vi "ABB measure Temperature.vi"(10 "Simulate":bool, 11 "Mode":enum16{"Initialise", "Read", "Close"}(ring)) -> (0 "error out":errorcluster, 2 "Reading strings":string[](array[string]), 3 "Readings":dbl[](array[numeric]))   [LabVIEW 2017]
uses:
  RTD Type.ctl
  TC Type.ctl
  <vilib>/DAQmx/read.llb/DAQmx Read (Analog 2D DBL NChan NSamp).vi
  <vilib>/Analysis/baseanly.llb/Mean (DBL).vi
  ABB global.vi
  <vilib>/DAQmx/create/channels.llb/DAQmx Create Channel (AI-Temperature-RTD).vi
  <vilib>/DAQmx/configure/timing.llb/DAQmx Timing (Sample Clock).vi
  <vilib>/DAQmx/create/channels.llb/DAQmx Create Channel (AI-Temperature-Thermocouple).vi
  <vilib>/DAQmx/miscellaneous.llb/DAQmx Fill In Error Info.vi
  <resource>/objmgr/daqmx.rc
  <vilib>/Analysis/NI_AALBase.lvlib
panel:
  out "error out 2":errorcluster
  out "AvailSampPerChan":u32
  out "RT resistance":dbl[](array[numeric])
  out "RT types":i32[](array[numeric])
  out "TC Types":i32[](array[numeric])
  in  "Thermocouple Type":T1 items=["J", "K", "N", "R", "S", "T", "B", "E"]
  in  "RTD Type":T2 items=["PT100 3W", "PT100 4W", "PT1000 3W", "PT1000 4W"]
  out "Array":string[](array[string])
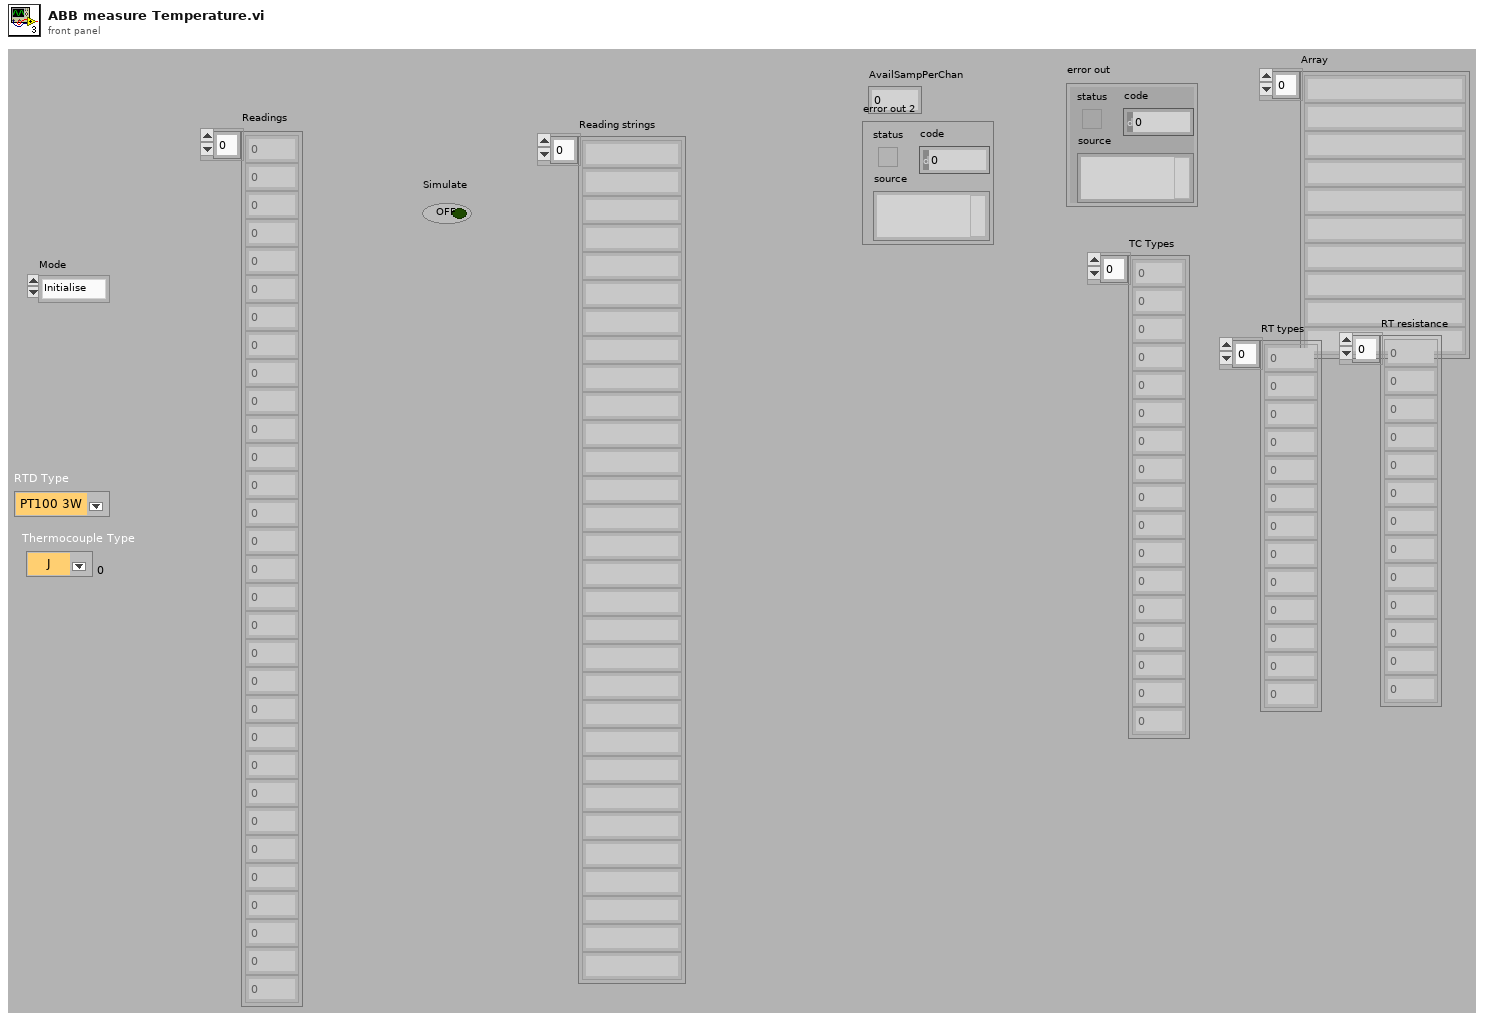
[diagram p1: front panel]
types:
  T1 = typedef "TC Type.ctl" = u16
  T2 = typedef "RTD Type.ctl" = u16
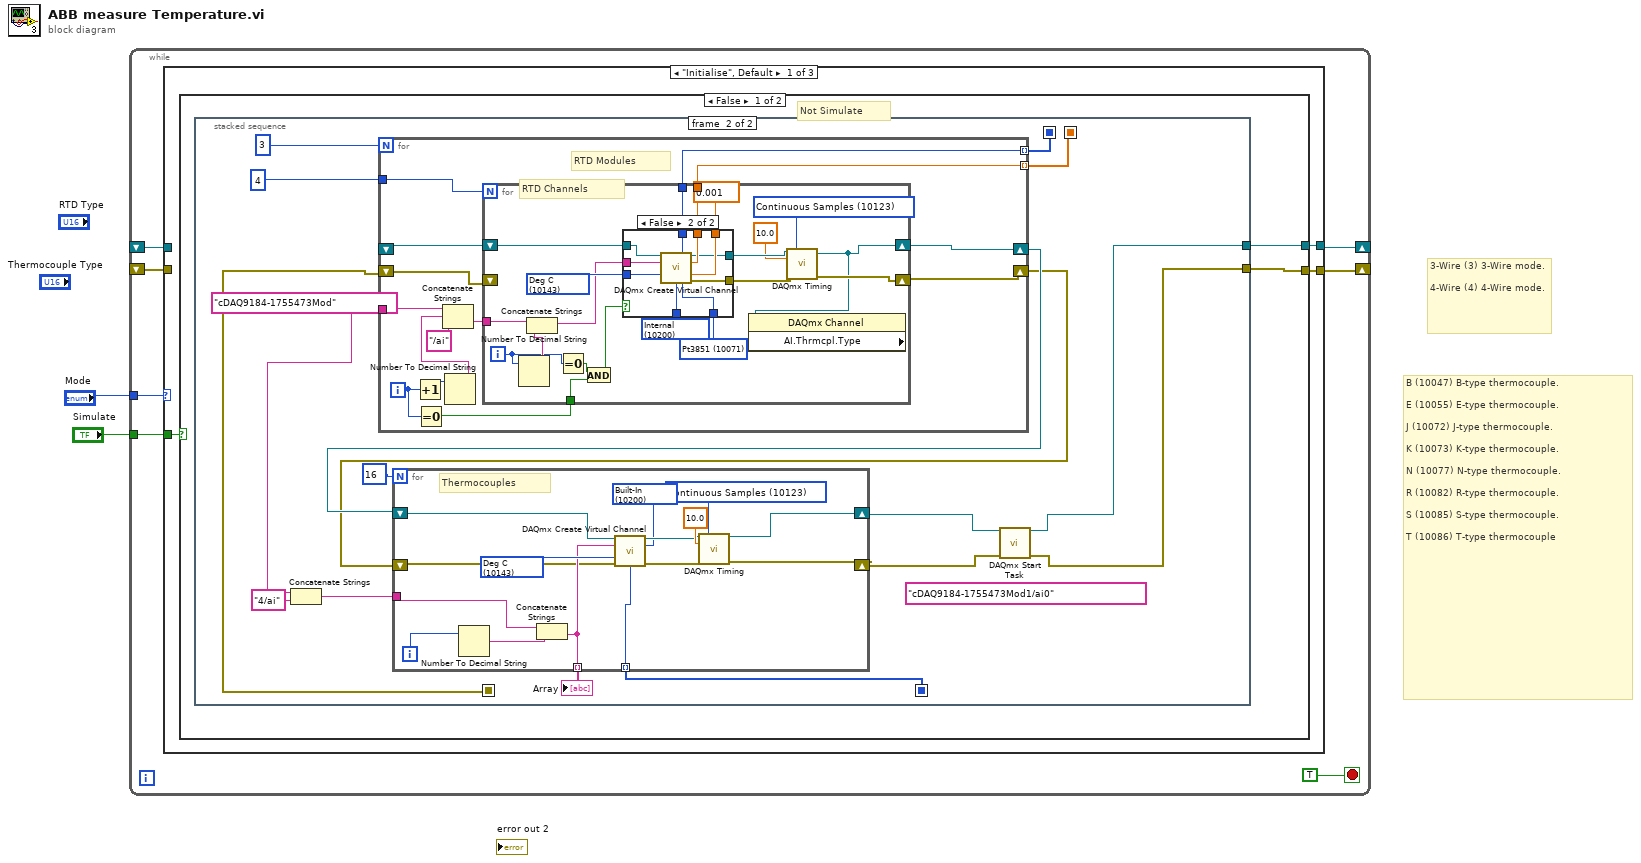
[diagram p0: block diagram]
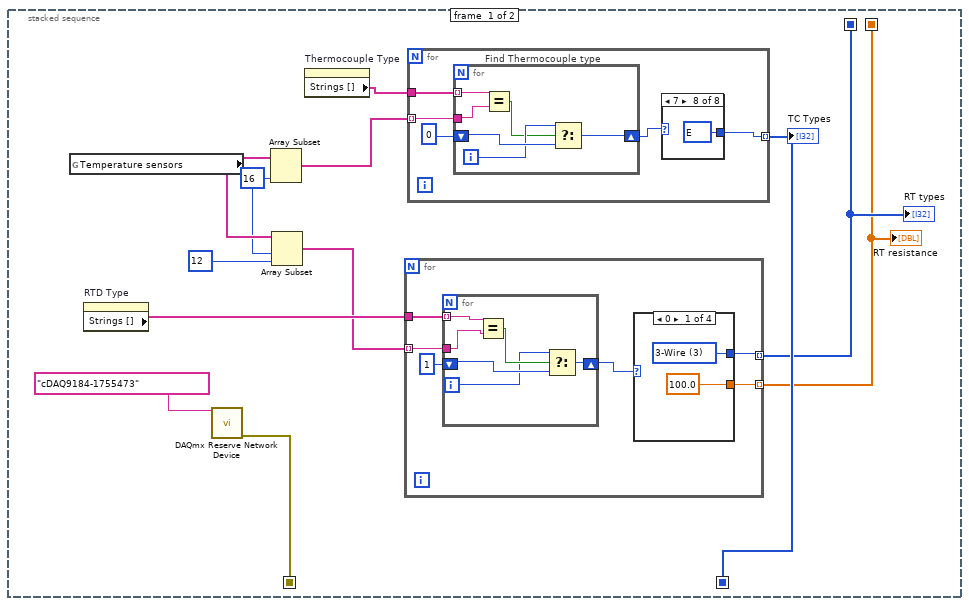
[diagram p2: hidden frame]
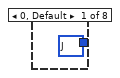
[diagram p3: hidden frame]
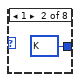
[diagram p4: hidden frame]
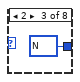
[diagram p5: hidden frame]
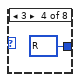
[diagram p6: hidden frame]
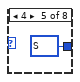
[diagram p7: hidden frame]
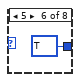
[diagram p8: hidden frame]
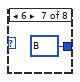
[diagram p9: hidden frame]
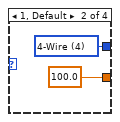
[diagram p10: hidden frame]
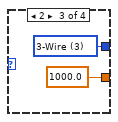
[diagram p11: hidden frame]
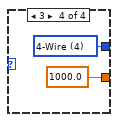
[diagram p12: hidden frame]
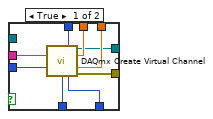
[diagram p13: hidden frame]
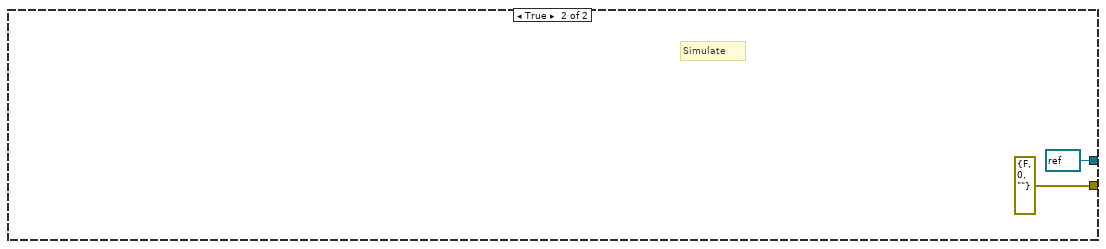
[diagram p14: hidden frame]
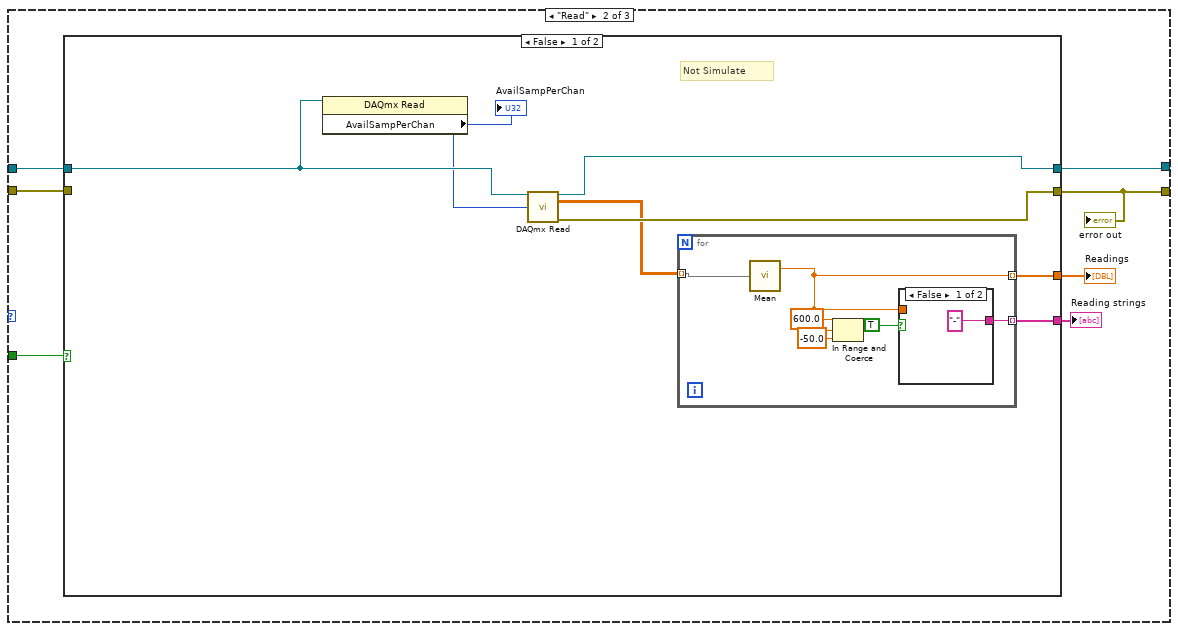
[diagram p15: hidden frame]
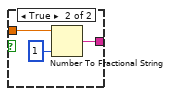
[diagram p16: hidden frame]
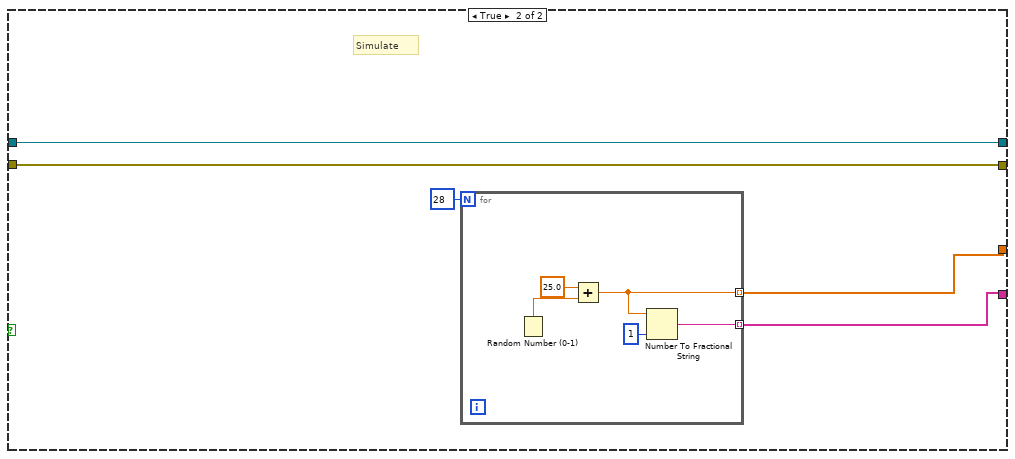
[diagram p17: hidden frame]
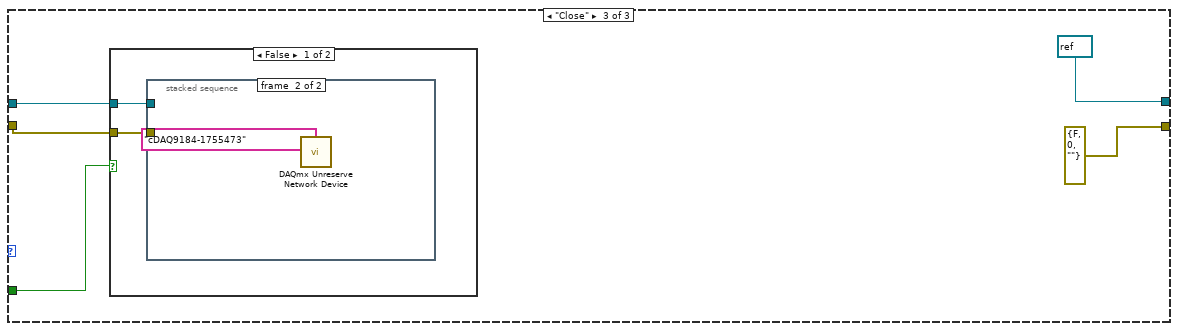
[diagram p18: hidden frame]
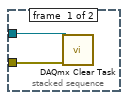
[diagram p19: hidden frame]
diagram:
  # "3-Wire (3) 3-Wire mode. \n \n4-Wire (4) 4-Wire mode."
  # "B (10047) B-type thermocouple. \n \nE (10055) E-type thermocouple. \n \nJ (10072) J-type thermocouple. \n \nK (10073) K-type thermocouple. \n \nN (10077) N-type thermocouple. \n \nR (10082) R-type thermocouple. \n \nS (10085) S-type thermocouple. \n \nT (10086) T-type thermocouple"
  n1 = while {
    tunnel: "Mode" -> [w9]
    shift-right: [w4] -> _
    shift-left: _ -> [w7]
    shift-right: [w5] -> _
    shift-left: _ -> [w6]
    tunnel: "Simulate" -> [w3]
    stop <- TRUE stop-if-true
    n2 = case shown="\"Initialise\", Default" w9 {
      tunnel: [w12 w159 refnum<k21> refnum ("task out")] -> w4
      tunnel: [w11 w154 errorcluster {"status"=FALSE, "code"=0, "source"=""} ("error out")] -> w5
      tunnel: w7 -> [_ w158 w191]
      tunnel: w6 -> [_ w157 w188]
      tunnel: w3 -> [w10 w156 w187]
      frame "Initialise", Default {
        n3 = case shown="False" w10 {
          tunnel: [w14 refnum<k21> refnum ("task out")] -> w12
          tunnel: [w13 errorcluster {"status"=FALSE, "code"=0, "source"=""} ("error out")] -> w11
          frame False {
            # "Not Simulate"
            n4 = stacked-sequence {
              seq-local: [w21 _] -> [_ w66]
              seq-local: [w18 _] -> [_ w72]
              seq-local: [w17 _] -> [_ w73]
              seq-local: [w15 _] -> [_ w67]
              tunnel: [_ w68] -> w14
              tunnel: [_ w69] -> w13
              frame #0 {
                w25 = 16 ("length")
                n5 = global read "ABB global.vi" "Temperature sensors"() -> (w26:string[])
                n6 = property on="RTD Type" class="Ring (strict)"() -> ("Strings []"=w20:string[])  [unwired: 2 in, 2 out]
                n7 = call <vilib>:"DAQmx Reserve Network Device.vi"("device in"=tag "cDAQ9184-1755473") -> ("error out"=w15:errorcluster)  [unwired: 13 in, 1 out]
                n8 = Array Subset(array=w26, length=w25) -> (w23:string[])  [unwired: 1 in]
                n9 = Array Subset(array=w26, index=w25, length=12) -> (w19:string[])
                n10 = property on="Thermocouple Type" class="Ring (strict)"() -> ("Strings []"=w22:string[])  [unwired: 2 in, 2 out]
                n11 = for {
                  tunnel: w20 -> [w51]
                  tunnel: w19 -> [w50] mode=indexing
                  tunnel: [w48] -> w18 mode=indexing
                  tunnel: [w47] -> w17 mode=indexing
                  n12 = for {
                    tunnel: w51 -> [w64] mode=indexing
                    tunnel: w50 -> [w63]
                    shift-right: [w61] -> w49
                    shift-left: 1 -> [w62]
                    i -> [w60]
                    n13 = Equal?(x=w64, y=w63) -> (x = y?=w65:bool)
                    n14 = Select(t=w60, s=w65, f=w62) -> (s? t:f=w61:i32)
                  }
                  n15 = case shown="0" w49 {
                    tunnel: [w53 w55 w57 w59] -> w48
                    tunnel: [100.0 100.0 1000.0 1000.0] -> w47
                    frame 0 {
                      w53 = 3 items=["2-Wire"=2, "3-Wire"=3, "4-Wire"=4] ("resistance configuration")
                    }
                    frame 1, Default {
                      w55 = 4 items=["2-Wire"=2, "3-Wire"=3, "4-Wire"=4] ("resistance configuration")
                    }
                    frame 2 {
                      w57 = 3 items=["2-Wire"=2, "3-Wire"=3, "4-Wire"=4] ("resistance configuration")
                    }
                    frame 3 {
                      w59 = 4 items=["2-Wire"=2, "3-Wire"=3, "4-Wire"=4] ("resistance configuration")
                    }
                  }
                }
                "RT types" <- w18
                "RT resistance" <- w17
                n16 = for {
                  tunnel: w23 -> [w30] mode=indexing
                  tunnel: w22 -> [w31]
                  tunnel: [w27] -> w21 mode=indexing
                  # "Find Thermocouple type"
                  n17 = for {
                    tunnel: w31 -> [w45] mode=indexing
                    tunnel: w30 -> [w44]
                    shift-right: [w40] -> w28
                    shift-left: 0 -> [w43]
                    i -> [w42]
                    n18 = Equal?(x=w45, y=w44) -> (x = y?=w41:bool)
                    n19 = Select(t=w42, s=w41, f=w43) -> (s? t:f=w40:i32)
                  }
                  n20 = case shown="7" w28 {
                    tunnel: [w32 w33 w34 w35 w36 w37 w38 w39] -> w27
                    frame 0, Default {
                      w32 = 10072 items=["J"=10072, "K"=10073, "N"=10077, "R"=10082, "S"=10085, "T"=10086, "B"=10047, "E"=10055] ("thermocouple type")
                    }
                    frame 1 {
                      w33 = 10073 items=["J"=10072, "K"=10073, "N"=10077, "R"=10082, "S"=10085, "T"=10086, "B"=10047, "E"=10055] ("thermocouple type")
                    }
                    frame 2 {
                      w34 = 10077 items=["J"=10072, "K"=10073, "N"=10077, "R"=10082, "S"=10085, "T"=10086, "B"=10047, "E"=10055] ("thermocouple type")
                    }
                    frame 3 {
                      w35 = 10082 items=["J"=10072, "K"=10073, "N"=10077, "R"=10082, "S"=10085, "T"=10086, "B"=10047, "E"=10055] ("thermocouple type")
                    }
                    frame 4 {
                      w36 = 10085 items=["J"=10072, "K"=10073, "N"=10077, "R"=10082, "S"=10085, "T"=10086, "B"=10047, "E"=10055] ("thermocouple type")
                    }
                    frame 5 {
                      w37 = 10086 items=["J"=10072, "K"=10073, "N"=10077, "R"=10082, "S"=10085, "T"=10086, "B"=10047, "E"=10055] ("thermocouple type")
                    }
                    frame 6 {
                      w38 = 10047 items=["J"=10072, "K"=10073, "N"=10077, "R"=10082, "S"=10085, "T"=10086, "B"=10047, "E"=10055] ("thermocouple type")
                    }
                    frame 7 {
                      w39 = 10055 items=["J"=10072, "K"=10073, "N"=10077, "R"=10082, "S"=10085, "T"=10086, "B"=10047, "E"=10055] ("thermocouple type")
                    }
                  }
                }
                "TC Types" <- w21
              }
              frame #1 {
                w77 = "cDAQ9184-1755473Mod"
                (unwired) tag "cDAQ9184-1755473Mod1/ai0" ("physical channels")
                n21 = Concatenate Strings(w77, "4/ai" ("string")) -> (w75:string)
                n22 = for {
                  N: 3 -> [_]
                  tunnel: 4 -> [w111]
                  tunnel: w77 -> [w109]
                  shift-right: [w105] -> w79
                  shift-left: _ -> [w104]
                  shift-right: [w101] -> w78
                  shift-left: w67 -> [w100]
                  tunnel: w73 -> [w99] mode=indexing
                  tunnel: w72 -> [w98] mode=indexing
                  i -> [w103]
                  # "RTD Modules"
                  n23 = Increment(x=w103) -> (x+1=w110:i32)
                  n24 = Equal To 0?(x=w103) -> (x = 0?=w102:bool)
                  n25 = Number To Decimal String(number=w110) -> (decimal integer string=w108:string)  [unwired: 1 in]
                  n26 = Concatenate Strings(w109, w108, "/ai" ("string")) -> (w106:string)
                  n27 = for {
                    N: w111 -> [_]
                    tunnel: w106 -> [w127]
                    shift-right: [w119] -> w105
                    shift-left: w104 -> [w114]
                    tunnel: w102 -> [w116]
                    shift-right: [w121] -> w101
                    shift-left: w100 -> [_]
                    tunnel: w99 -> [w113]
                    tunnel: w98 -> [w112]
                    i -> [w118]
                    w122 = 10123 items=["Finite Samples"=10178, "Continuous Samples"=10123, "Hardware Timed Single Point"=12522] ("sample mode")
                    w128 = 10143 items=["Deg C"=10143, "Deg F"=10144, "Kelvins"=10325, "Deg R"=10145, "From Custom Scale"=10065] ("units")
                    w129 = 10071 items=["Pt3750"=12481, "Pt3851"=10071, "Pt3911"=12482, "Pt3916"=10069, "Pt3920"=10053, "Pt3928"=12483, "Custom"=10137] ("rtd type")
                    w130 = 10200 items=["Internal"=10200, "External"=10167, "None"=10230] ("current excitation source")
                    # "RTD Channels"
                    n28 = Number To Decimal String(number=w118) -> (decimal integer string=w126:string)  [unwired: 1 in]
                    n29 = Concatenate Strings(w127, w126) -> (w120:string)
                    n30 = Equal To 0?(x=w118) -> (x = 0?=w117:bool)
                    n31 = And(x=w117, y=w116) -> (x .and. y?=w115:bool)
                    n32 = case shown="False" w115 {
                      tunnel: 0.001 ("current excitation value") -> [w140 w150]
                      tunnel: w113 -> [w139 w149]
                      tunnel: w130 -> [w138 w148]
                      tunnel: w129 -> [w137 w147]
                      tunnel: w128 -> [w136 w146]
                      tunnel: w112 -> [w135 w145]
                      tunnel: [w134 w144] -> w125
                      tunnel: [w133 w143] -> w124
                      tunnel: w120 -> [w132 w141]
                      tunnel: w114 -> [_ w142]
                      frame True {
                        n33 = call-poly <vilib>:"DAQmx Create Virtual Channel.vi"("resistance configuration"=w135, "physical channels"=w132, "r0"=w139, "units"=w136, "current excitation value"=w140, "current excitation source"=w138, "rtd type"=w137) -> ("task out"=w134:refnum<k21>, "error out"=w133:errorcluster)  [unwired: 7 in]
                      }
                      frame False {
                        n34 = call-poly <vilib>:"DAQmx Create Virtual Channel.vi"("task in"=w142, "resistance configuration"=w145, "physical channels"=w141, "r0"=w149, "units"=w146, "current excitation value"=w150, "current excitation source"=w148, "rtd type"=w147) -> ("task out"=w144:refnum<k21>, "error out"=w143:errorcluster)  [unwired: 6 in]
                      }
                    }
                    n35 = call-poly <vilib>:"DAQmx Timing.vi"("task/channels in"=w125, "sample mode"=w122, "rate"=10.0, "error in"=w124) -> ("task out"=w119:refnum<k21>, "error out"=w121:errorcluster)  [unwired: 10 in]
                    n36 = property class="DAQmx Channel" props=["AI.Thrmcpl.Type"](reference=w119) -> ()  [unwired: 1 in, 3 out]
                  }
                }
                n37 = for {
                  N: 16 -> [_]
                  shift-right: [w87] -> w71
                  shift-left: w79 -> [w84]
                  shift-right: [w86] -> w70
                  shift-left: w78 -> [w85]
                  tunnel: w75 -> [w90]
                  tunnel: [w88] -> w74 mode=indexing
                  tunnel: w66 -> [w83] mode=indexing
                  i -> [w92]
                  w89 = 10200 items=["Built-In"=10200, "Constant Value"=10116, "Channel"=10113] ("cjc source")
                  w97 = 10123 items=["Finite Samples"=10178, "Continuous Samples"=10123, "Hardware Timed Single Point"=12522] ("sample mode")
                  w93 = 10143 items=["Deg C"=10143, "Deg F"=10144, "Kelvins"=10325, "Deg R"=10145, "From Custom Scale"=10065] ("units")
                  # "Thermocouples"
                  n38 = Number To Decimal String(number=w92) -> (decimal integer string=w91:string)  [unwired: 1 in]
                  n39 = Concatenate Strings(w90, w91) -> (w88:string)
                  n40 = call-poly <vilib>:"DAQmx Create Virtual Channel.vi"("task in"=w84, "physical channels"=w88, "cjc source"=w89, "units"=w93, "error in"=w85, "thermocouple type"=w83) -> ("task out"=w94:refnum<k21>, "error out"=w95:errorcluster)  [unwired: 8 in]
                  n41 = call-poly <vilib>:"DAQmx Timing.vi"("task/channels in"=w94, "sample mode"=w97, "rate"=10.0, "error in"=w95) -> ("task out"=w87:refnum<k21>, "error out"=w86:errorcluster)  [unwired: 10 in]
                }
                "Array" <- w74
                n42 = call <vilib>:"DAQmx Start Task.vi"("task/channels in"=w71, "error in"=w70) -> ("task out"=w68:refnum<k21>, "error out"=w69:errorcluster)  [unwired: 12 in]
              }
            }
          }
          frame True {
            # "Simulate"
          }
        }
      }
      frame "Read" {
        n43 = case shown="False" w156 {
          tunnel: [w166 w181] -> w159
          tunnel: [w165 w180] -> w154
          tunnel: w158 -> [w164 w181]
          tunnel: w157 -> [_ w180]
          tunnel: [w161 w178] -> w155
          tunnel: [w160 w177] -> w153
          frame False {
            # "Not Simulate"
            n44 = property class="DAQmx Read"(reference=w164) -> ("AvailSampPerChan"=w163:u32)  [unwired: 1 in, 2 out]
            "AvailSampPerChan" <- w163
            n45 = call-poly <vilib>:"DAQmx Read.vi"("task/channels in"=w164, "number of samples per channel"=w163) -> ("task out"=w166:refnum<k21>, "data"=w162:dbl[][], "error out"=w165:errorcluster)  [unwired: 11 in]
            n46 = for {
              tunnel: w162 -> [w172] mode=indexing
              tunnel: [w169] -> w161 mode=indexing
              tunnel: [w168] -> w160 mode=indexing
              n47 = call-poly <vilib>:"Mean.vi"("X"=w172) -> ("mean"=w169:dbl)  [unwired: 1 out]
              n48 = In Range and Coerce(upper limit=600.0, x=w169, lower limit=-50.0) -> ()  [unwired: 2 out]
              n49 = case shown="False" TRUE {
                tunnel: w169 -> [_ w176]
                tunnel: ["-" w174] -> w168
                frame False {
                }
                frame True {
                  n50 = Number To Fractional String(number=w176, precision (6)=i16 1) -> (F-format string=w174:string)  [unwired: 2 in]
                }
              }
            }
          }
          frame True {
            # "Simulate"
            n51 = for {
              N: 28 -> [_]
              tunnel: [w184] -> w178 mode=indexing
              tunnel: [w182] -> w177 mode=indexing
              n52 = Random Number (0-1)() -> (number: 0 to 1=w186:dbl)
              n53 = Add(x=25.0, y=w186) -> (x+y=w184:dbl)
              n54 = Number To Fractional String(number=w184, precision (6)=i16 1) -> (F-format string=w182:string)  [unwired: 2 in]
            }
          }
        }
        "Readings" <- w155
        "error out" <- w154
        "Reading strings" <- w153
      }
      frame "Close" {
        n55 = case shown="False" w187 {
          tunnel: w191 -> [w193 _]
          tunnel: w188 -> [w192 _]
          frame False {
            n56 = stacked-sequence {
              tunnel: w193 -> [w195 _]
              tunnel: w192 -> [w194 _]
              frame #0 {
                n57 = call <vilib>:"DAQmx Clear Task.vi"("task in"=w195, "error in"=w194) -> ()  [unwired: 13 in, 1 out]
              }
              frame #1 {
                n58 = call <vilib>:"DAQmx Unreserve Network Device.vi"("device in"=tag "cDAQ9184-1755473") -> ()  [unwired: 13 in, 2 out]
              }
            }
          }
          frame True {
          }
        }
      }
    }
  }
